vi "Downsample FFT.vi"(1 "Samples/Symbol":i32, 2 "FFT Received":cdb[](array[numeric])) -> (0 "FFT Downsampled":cdb[](array[numeric]))   [LabVIEW 2018]
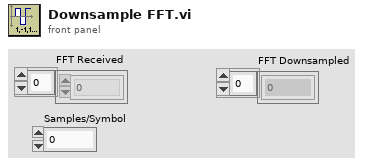
[diagram p1: front panel]
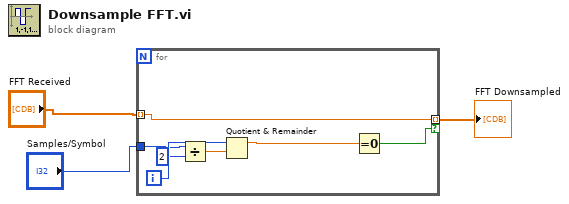
[diagram p0: block diagram]
diagram:
  n1 = for {
    tunnel: "FFT Received" -> [w9] mode=indexing
    tunnel: "Samples/Symbol" -> [w5]
    tunnel: [w9] -> w1 mode=indexing if=w8
    i -> [w10]
    n2 = Divide(x=w5, y=2) -> (x/y=w6:dbl)
    n3 = Quotient & Remainder(x=w10, y=w6) -> (x-y*floor(x/y)=w7:dbl)  [unwired: 1 out]
    n4 = Equal To 0?(x=w7) -> (x = 0?=w8:bool)
  }
  "FFT Downsampled" <- w1
